vi "SSC Digital Calculate Per-Instrument Per-Site to Per-Site LUT.vi"(0 "Digital SSC In":T2[](array[typedef]), 7 "Sites":i32[](array[numeric])) -> (4 "Per-Instrument Per-Site to Per-Site LUT":T1[](array[typedef]))   [LabVIEW 2020]
uses:
  SSC Digital/SSC Digital.ctl
  Digital 1D Location Array in a Cluster.ctl
  Shared SubVIs/Trim Whitespace [Inlined].vi
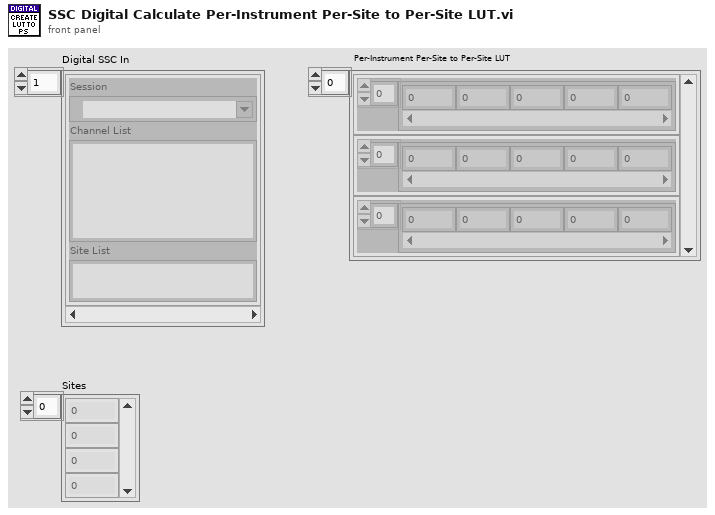
[diagram p1: front panel]
types:
  T1 = typedef "Digital 1D Location Array in a Cluster.ctl" = cluster{"Digital 1D Location Array":i32[]}
  T2 = typedef "SSC Digital.ctl" = cluster{"Session":refnum<k15>, "Channel List":string, "Site List":string}
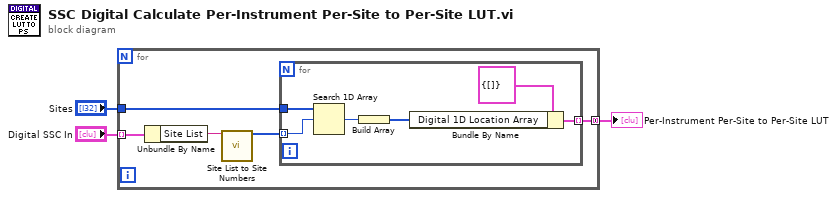
[diagram p0: block diagram]
diagram:
  n1 = for {
    tunnel: "Digital SSC In" -> [w8] mode=indexing
    tunnel: "Sites" -> [w7]
    tunnel: [w4] -> w1 mode=concatenating
    n2 = Unbundle By Name(w8) -> ("Site List"=w6:string)
    n3 = call "Site List to Site Numbers.vi"("Site List"=w6) -> ("Site Numbers"=w5:i32[])  [unwired: 13 in, 1 out]
    n4 = for {
      tunnel: w5 -> [w13] mode=indexing
      tunnel: w7 -> [w14]
      tunnel: [w9] -> w4 mode=indexing
      n5 = Search 1D Array(1D array=w14, element=w13) -> (index of element=w12:i32)  [unwired: 1 in]
      n6 = Build Array(w12) -> (w10:i32[])
      n7 = Bundle By Name(cluster=T1 {"Digital 1D Location Array"=[]} ("Digital 1D Location Array in a Cluster"), "Digital 1D Location Array"=w10) -> (w9:T1)
    }
  }
  "Per-Instrument Per-Site to Per-Site LUT" <- w1
